vi "Analog DAQ-Core_Initialize.vi"(0 "Initialization Sequence":string, 5 "FTW Actor Instance Configuration":string, 11 "error in (no error)":errorcluster) -> (4 "Actor Template-Core out":refnum<class "Analog DAQ-Core.lvclass">, 6 "Incoming Requests":refnum<event-registration>, 8 "Local Messages":refnum<event-registration>, 15 "error out":errorcluster)   [LabVIEW 2013, in "Analog DAQ-Core.lvclass"]
uses:
  Analog DAQ-Core.lvclass
  source/actor/Message/Request/FTW-Message-IncomingRequest.lvclass
  source/actor/Message/Base/FTW-Message.lvclass
  Analog DAQ-Core.lvclass/Analog DAQ-Core.ctl
  source/Reflection/FTW-Reflection-Type.vi
  source/JSON/FTW-JSON-Core-LibraryFilepath.vi
  source/JSON/FTW-JSON-Core-GetFlattenedValue.vi
  source/JSON/FTW-JSON-Core-LibraryError.vi
  source/CodeGen/JSON Deserialize/FTW-JSON-Deserialize.xnode
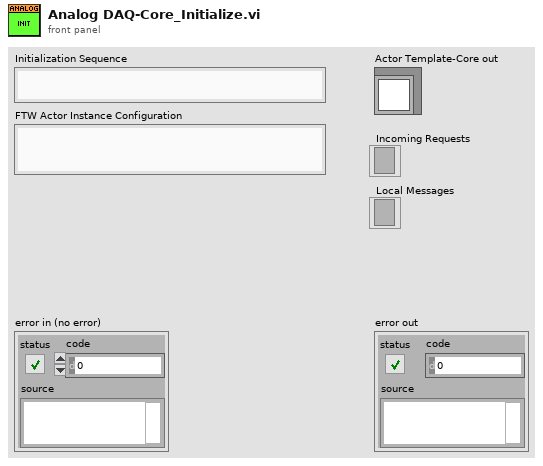
[diagram p1: front panel]
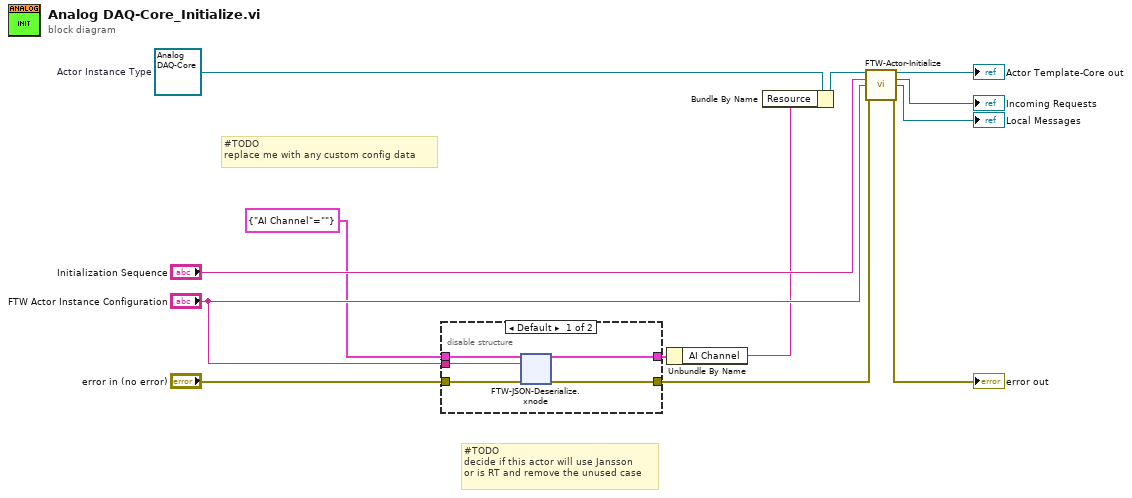
[diagram p0: block diagram]
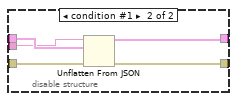
[diagram p2: hidden frame]
diagram:
  w11 = refnum<class "Analog DAQ-Core.lvclass"> refnum  # Actor Instance Type
  # "#TODO\ndecide if this actor will use Jansson\nor is RT and remove the unused case"
  # "#TODO\nreplace me with any custom config data"
  n1 = disable-structure shown="Default" {
    disable-tunnel: "error in (no error)" -> [w18 w57]
    disable-tunnel: [w17 w56] -> w7
    disable-tunnel: "FTW Actor Instance Configuration" -> [w16 w54]
    disable-tunnel: cluster{"AI Channel":string} {"AI Channel"=""} ("Type and Defaults") -> [w15 w55]
    disable-tunnel: [w14 w53] -> w3
    frame condition #0 (active) {
      n2 = xnode "FTW-JSON-Deserialize.xnode"("Type and Defaults"=w15, "JSON String"=w16, "error in"=w18) -> ("Values"=w14:cluster{"AI Channel":string}, "error out"=w17:errorcluster)
    }
    frame condition #1 {
      n3 = Unflatten From JSON(JSON string=w54, type and defaults=w55, error in (no error)=w57) -> (value=w53:cluster{"AI Channel":string}, error out=w56:errorcluster)  [unwired: 4 in]
    }
  }
  n4 = Unbundle By Name(w3) -> ("AI Channel"=w2:string)
  n5 = Bundle By Name(cluster=w11, "Resource"=w2) -> (w4:refnum<class "Analog DAQ-Core.lvclass">)
  n6 = call-dynamic "FTW-Actor-Initialize.vi"("FTW Actor Instance Type"=w4, "Initialization Job Sequence"="Initialization Sequence", "Actor Instance Configuration"="FTW Actor Instance Configuration", "error in"=w7) -> ("FTW Actor Instance"=→"Actor Template-Core out":refnum<class "Analog DAQ-Core.lvclass">, "Incoming Requests"=→"Incoming Requests":refnum<event-registration>, "Local Messages"=→"Local Messages":refnum<event-registration>, "error out"=→"error out":errorcluster)  [unwired: 8 in]
